vi "Main.vi"() -> ()   [LabVIEW 2015, in "Thermal Chamber Controller_DQMH.lvlib"]
doc: "This application is based on the Delacor QMH project template. Run this VI directly to test the module in stand alone mode. Run the module tester VI to test the module in external launch mode.\n\nThis example implements a Thermal Chamber Controller with a singleton Delacor QMH module.\n\n_____\nBased on Delacor QMH Project Template 3.0.\nReviewed and updated to match QMH Project Template 4.0.\n<b>Note:</b> This VI was modified by the <b>Validate DQMH Module</b> tool to upgrade it to the DQMH 3.0 implementation of the 'Show Diagram' message, which checks the password-protected status of the Main VI before showing the diagram.\n____\nDelacor QMH Thermal Chamber Examples 4.0.0.21\nCopyright (c) 2018, Delacor"
uses:
  Thermal Chamber Controller_DQMH.lvlib
  <vilib>/Delacor/Delacor QMH/Libraries/Module Admin_class/Delacor_lib_QMH_Module Admin.lvclass
  Module Data--cluster.ctl
  Heater State--enum.ctl
  Update Set Point Argument--cluster.ctl
  Update Ramp Rate Argument--cluster.ctl
  Update Heater State Argument--cluster.ctl
  Request and Wait for Status Argument--cluster.ctl
  Request and Wait for Status (Reply Payload)--cluster.ctl
  Stop Argument--cluster.ctl
  <vilib>/Delacor/Delacor QMH/Libraries/Module Admin_class/Delacor_lib_QMH_Module Admin.lvclass/Delacor_lib_QMH_Module Admin.ctl
  <vilib>/Delacor/Delacor QMH/Libraries/Module Admin_class/Delacor_lib_QMH_Get External Launch.vi
  <vilib>/Delacor/Delacor QMH/Libraries/Message Queue_class/Delacor_lib_QMH_Enqueue Message (Single).vi
  <vilib>/Utility/error.llb/Error Cluster From Error Code.vi
  <vilib>/ErrorRing/Error Ring.xnode
  <vilib>/Delacor/Delacor QMH/Libraries/Message Queue_class/Delacor_lib_QMH_Message Queue.lvclass
  Thermal Chamber Response Simulator/Thermal Chamber Response Simulator.lvlib
panel:
  in  "Enable Heater":bool
  in  "Disable Heater":bool
  in  "Ramp Rate (deg C / second)":dbl=1.0
  in  "Temperature Set Point (deg C)":dbl=22.0
  out "Heater State":bool
  out "Actual Temperature":dbl format="%.2f"
  out "Chamber Temperature Chart":T1(graph)
  in  "Simulate MHL Error":bool
  in  "Simulate EHL Error":bool
  out "error out":errorcluster
  in  "Module Admin":refnum<class "Delacor_lib_QMH_Module Admin.lvclass">
  out "Status":string
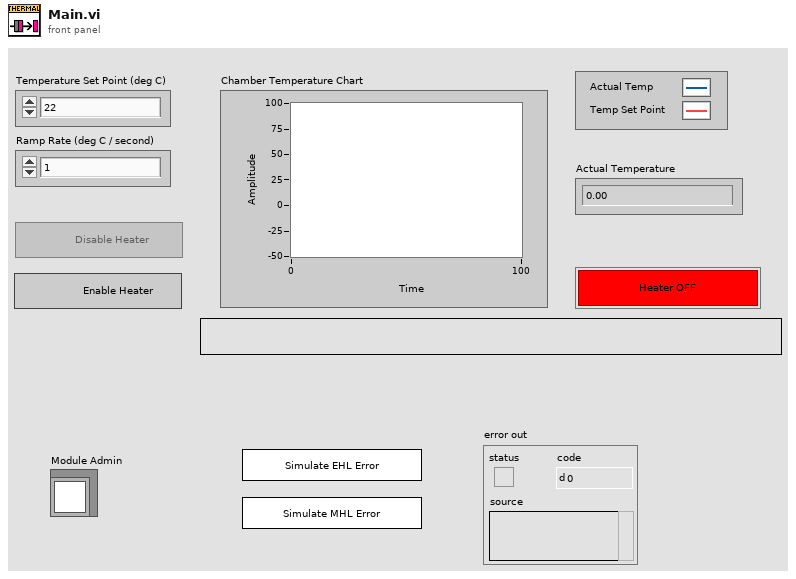
[diagram p1: front panel]
types:
  T1 = cluster{"Actual Temperature":dbl, "Required Temperature deg C":dbl}
  T2 = typedef "Thermal Chamber Controller_DQMH.lvlib/Request Events--cluster.ctl" = cluster{"Stop Module":refnum<user-event>, "Show Panel":refnum<user-event>, "Hide Panel":refnum<user-event>, "Get Module Execution Status":refnum<user-event>, "Show Diagram":refnum<user-event>, "Update Set Point":refnum<user-event>, "Update Ramp Rate":refnum<user-event>, "Update Heater State":refnum<user-event>, "Update Chamber Status":refnum<user-event>, "Request and Wait for Status":refnum<user-event>}
  T3 = typedef "Thermal Chamber Controller_DQMH.lvlib/Module Data--cluster.ctl" = cluster{"Status":string, "Temperature Set Point":dbl, "Temperature Ramp Rate":dbl, "Heater State":T4, "Disable Heater ref":refnum<vi>, "Enable Heater ref":refnum<vi>, "Temperature Set Point (deg C) ref":refnum<vi>, "Temperature Ramp Rate (Deg C / sec) ref":refnum<vi>}
  T4 = typedef "Thermal Chamber Controller_DQMH.lvlib/Heater State--enum.ctl" = enum16{"Heater Enabled", "Heater Disabled"}
  T5 = typedef "Thermal Chamber Controller_DQMH.lvlib/Update Set Point Argument--cluster.ctl" = cluster{"Temperature Set Point":dbl}
  T6 = typedef "Thermal Chamber Controller_DQMH.lvlib/Update Ramp Rate Argument--cluster.ctl" = cluster{"Temperature Ramp Rate":dbl}
  T7 = typedef "Thermal Chamber Controller_DQMH.lvlib/Update Heater State Argument--cluster.ctl" = cluster{"Heater State":T4}
  T8 = typedef "Thermal Chamber Controller_DQMH.lvlib/Request and Wait for Status Argument--cluster.ctl" = cluster{"Wait Notifier":refnum<notifier>}
  T9 = enum32{"invalid lock state", "Not Locked", "Locked (No Password)", "Password-protected"}
  T10 = typedef "Thermal Chamber Controller_DQMH.lvlib/Stop Argument--cluster.ctl" = cluster{"Origin":string, "Exit via Stop Module Req?":bool, "Wait for Module to stop?":bool}
  T11 = enum32{"Invalid", "Standard", "Closed", "Hidden", "Minimized", "Maximized"}
  T12 = typedef "Thermal Chamber Controller_DQMH.lvlib/Request and Wait for Status (Reply Payload)--cluster.ctl" = cluster{"Actual Temperature":dbl, "Temperature Set Point":dbl, "Temperature Ramp Rate":dbl, "Heater State":T4, "error":errorcluster}
  T13 = cluster{"Actual Temperature":dbl, "Temperature Set Point (deg C)":dbl}
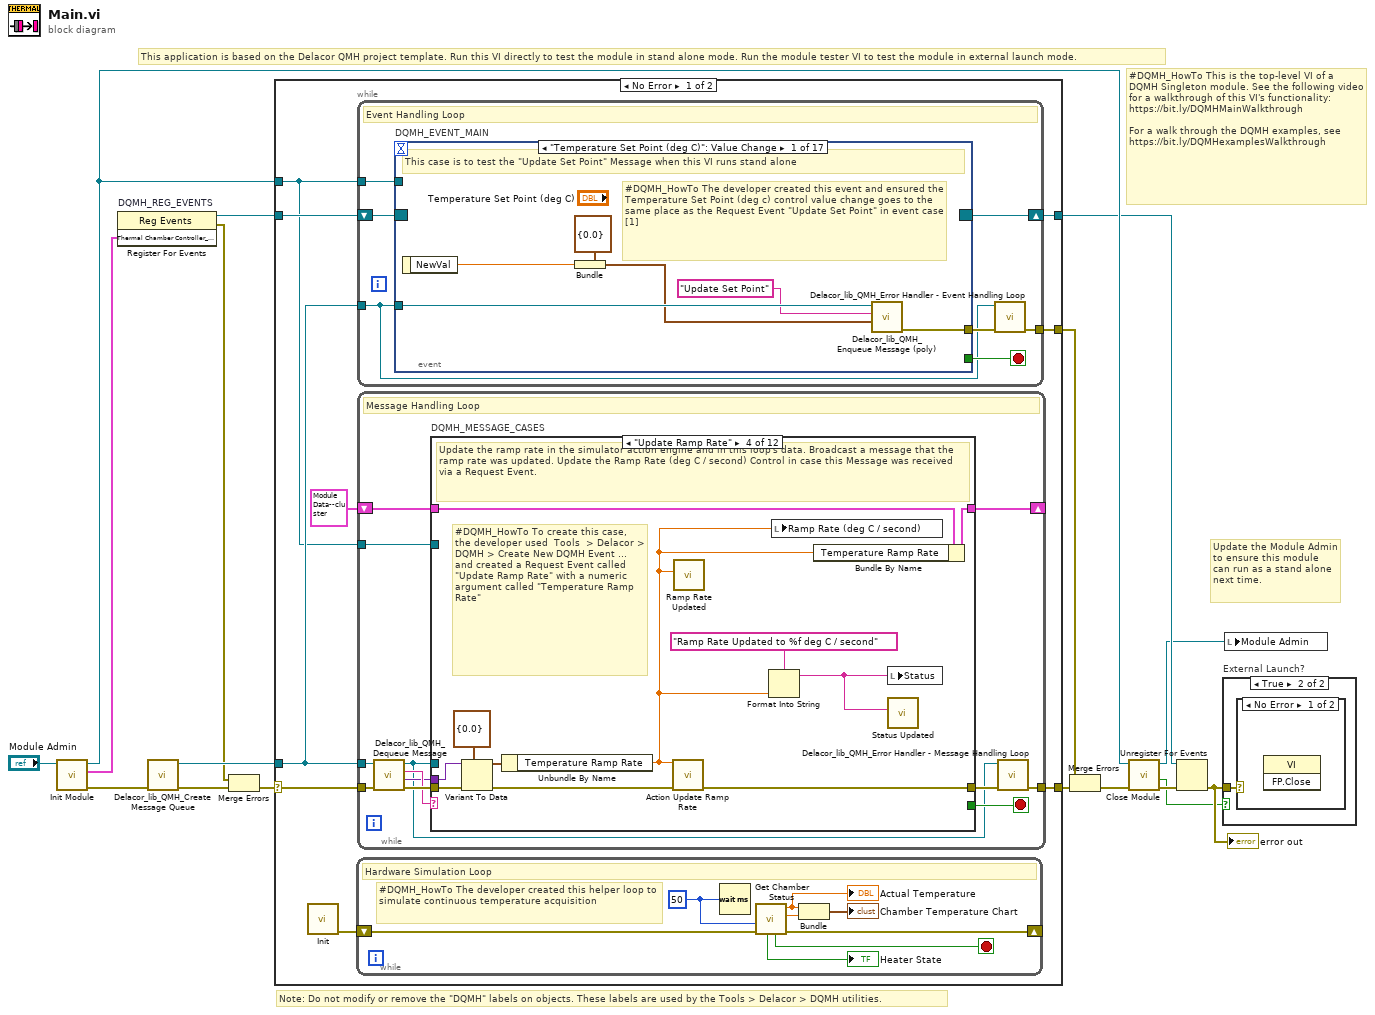
[diagram p0: block diagram]
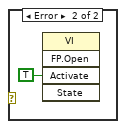
[diagram p3: hidden frame]
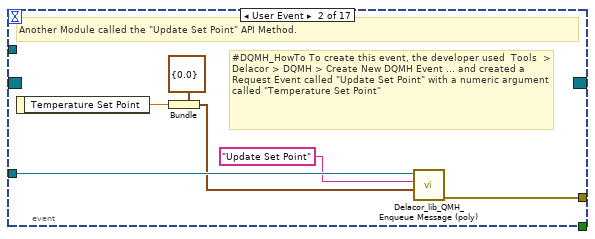
[diagram p4: hidden frame]
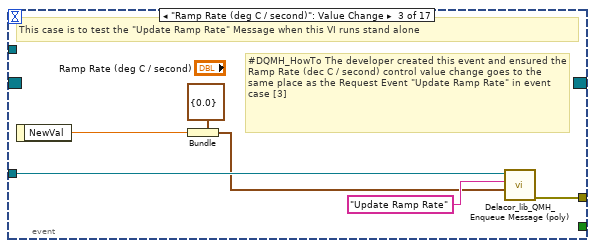
[diagram p5: hidden frame]
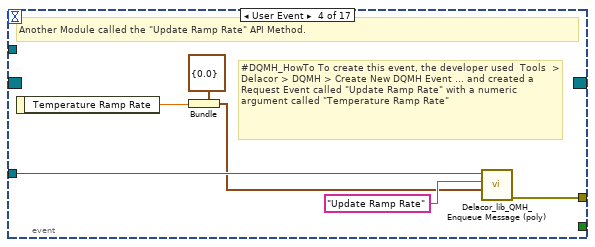
[diagram p6: hidden frame]
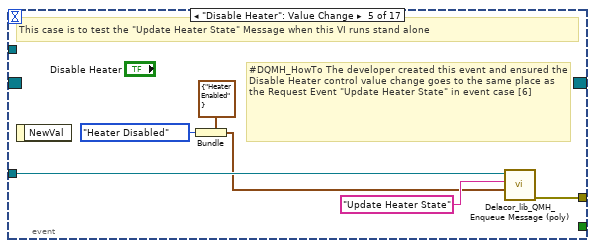
[diagram p7: hidden frame]
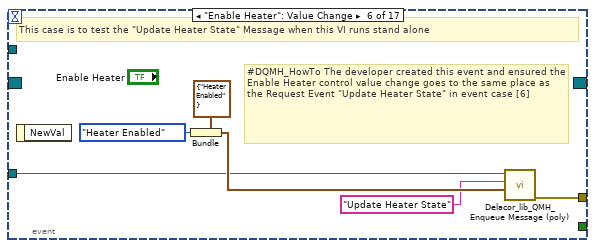
[diagram p8: hidden frame]
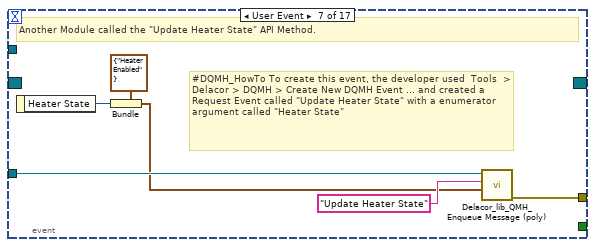
[diagram p9: hidden frame]
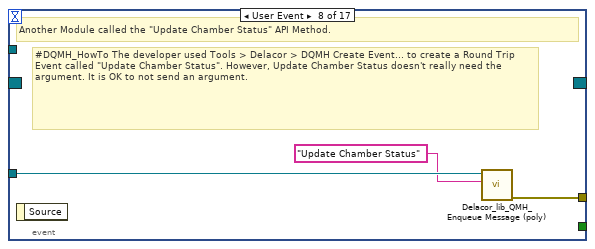
[diagram p10: hidden frame]
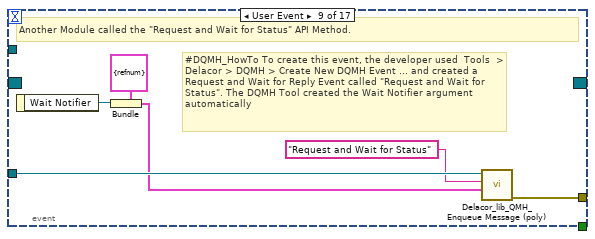
[diagram p11: hidden frame]
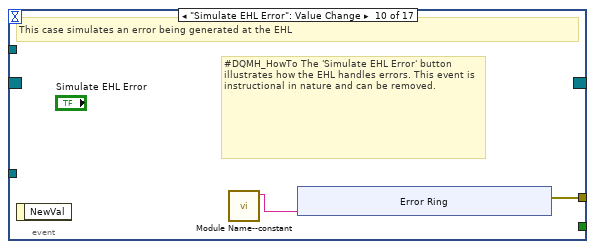
[diagram p12: hidden frame]
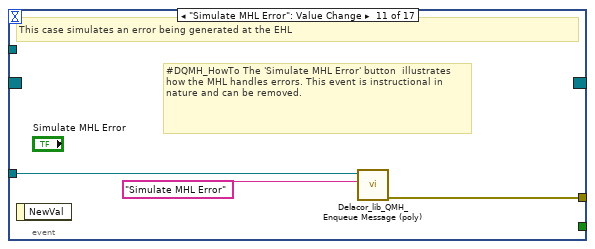
[diagram p13: hidden frame]
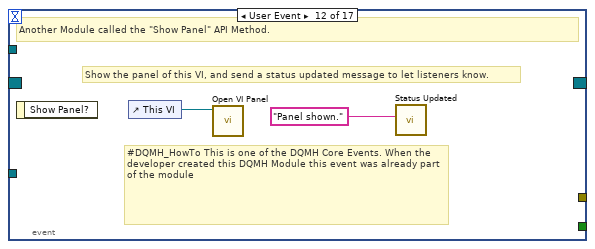
[diagram p14: hidden frame]
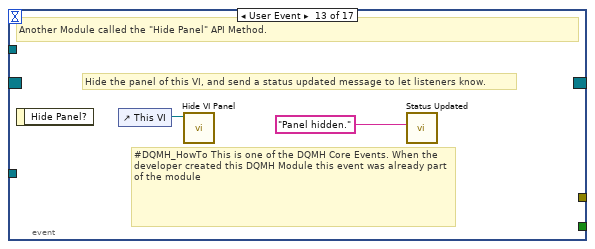
[diagram p15: hidden frame]
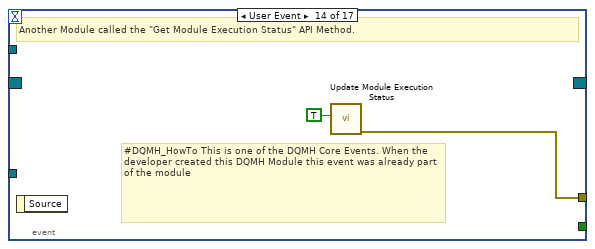
[diagram p16: hidden frame]
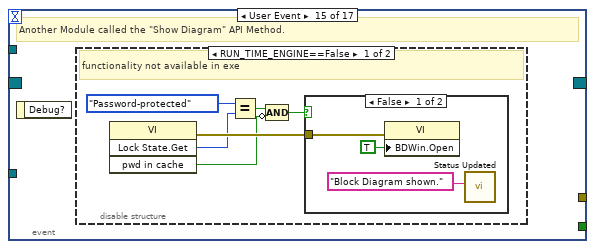
[diagram p17: hidden frame]
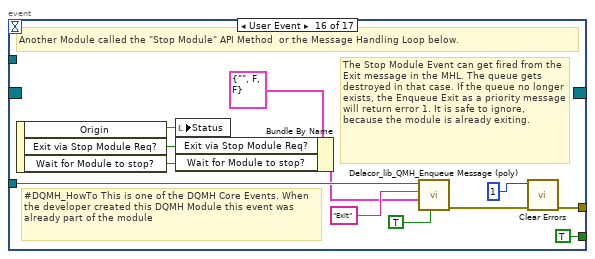
[diagram p20: hidden frame]
diagram:
  # "#DQMH_HowTo This is the top-level VI of a DQMH Singleton module. See the following video for a walkthrough of this VI's functionality: https://bit.ly/DQMHMainWalkthrough\n\nFor a walk through the DQMH examples, see https://bit.ly/DQMHexamplesWalkthrough"
  # "This application is based on the Delacor QMH project template. Run this VI directly to test the module in stand alone mode. Run the module tester VI to test the module in external launch mode."
  # "Note: Do not modify or remove the \"DQMH\" labels on objects. These labels are used by the Tools > Delacor > DQMH utilities."
  # "Update the Module Admin to ensure this module can run as a stand alone next time."
  n1 = call "Init Module.vi"("Singleton Module Admin in"="Module Admin") -> ("error out"=w15:errorcluster, "Thermal Chamber Controller_DQMH Request Events"=w12:T2, "Singleton Module Admin out"=w17:refnum<class "Delacor_lib_QMH_Module Admin.lvclass">)  [unwired: 8 in]
  n2 = register-events "DQMH_REG_EVENTS"(w12) -> (reference out=w13:refnum<event-registration>, error out=w1:errorcluster)  [unwired: 2 in]
  n3 = call <vilib>:"Delacor_lib_QMH_Create Message Queue.vi"("error in (no error)"=w15) -> ("error out"=w3:errorcluster, "Message Queue out"=w11:refnum<class "Delacor_lib_QMH_Message Queue.lvclass">)  [unwired: 9 in]
  n4 = Merge Errors(w1, w3) -> (w2:errorcluster)
  n5 = case shown="No Error" w2 {
    selector: w2 -> [w20 w314]
    tunnel: [w26 w314] -> w16
    tunnel: [w25 w319] -> w14
    tunnel: w13 -> [w23 w319]
    tunnel: w11 -> [w22 _]
    tunnel: [w21 _] -> w7
    tunnel: w17 -> [w19 w315]
    frame No Error {
      n6 = call "Init.vi"() -> ("error out"=w18:errorcluster)  [unwired: 11 in]
      n7 = while {
        shift-right: [w30] -> _
        shift-left: w18 -> [w33]
        stop <- w32 stop-if-true
        w34 = u32 50 ("millisecond multiple")
        # "#DQMH_HowTo The developer created this helper loop to simulate continuous temperature acquisition"
        # "Hardware Simulation Loop"
        n8 = Wait (ms)(milliseconds to wait=w34) -> ()  [unwired: 1 out]
        n9 = call "Get Chamber Status.vi"("error in (no error)"=w33, "Time Interval (ms)"=w34) -> ("error out"=w30:errorcluster, "Temperature Set Point (deg C)"=w31:dbl, "Actual Temperature"=w29:dbl, "Application Exit"=w32:bool, "Heater State"=→"Heater State":bool)  [unwired: 4 in, 1 out]
        "Actual Temperature" <- w29
        n10 = Bundle("Actual Temperature"=w29, "Temperature Set Point (deg C)"=w31) -> (→"Chamber Temperature Chart":T13)  [unwired: 1 in]
      }
      n11 = while {
        tunnel: w22 -> [w35]
        shift-right: [w40] -> w25
        shift-left: w23 -> [w41]
        tunnel: [w37] -> w21
        tunnel: w19 -> [w36]
        stop <- w38 stop-if-true
        # "Event Handling Loop"
        n12 = event "DQMH_EVENT_MAIN" shown="[0] \"Temperature Set Point (deg C)\": Value Change" {
          selector: w41 -> [_ _ _ _ _ _ _ _ _ _ _ _ _ _ _ _ _]
          dyn-events: [_ _ _ _ _ _ _ _ _ _ _ _ _ _ _ _ _] -> w40
          timeout: _ -> [_ _ _ _ _ _ _ _ _ _ _ _ _ _ _ _ _]
          tunnel: [_ _ _ _ _ _ _ _ _ _ _ _ _ _ _ TRUE ("Discard?") _] -> w38
          tunnel: w35 -> [w47 w53 w56 w65 w69 w74 w83 w86 w92 _ w104 _ _ _ _ w129 w132]
          tunnel: [w42 w49 w55 w61 w68 w73 w79 w84 w88 w94 w102 _ _ w110 _ w124 w134] -> w39
          tunnel: w36 -> [_ _ _ _ _ _ _ _ _ _ _ _ _ _ _ _ w135]
          event "Temperature Set Point (deg C)": Value Change {
            # "#DQMH_HowTo The developer created this event and ensured the Temperature Set Point (deg c) control value change goes to the same place as the Request Event \"Update Set Point\" in event case [1]"
            # "This case is to test the \"Update Set Point\" Message when this VI runs stand alone"
            n13 = event-data() -> ("NewVal"=w43:dbl)  [unwired: 1 in]
            n14 = Bundle(cluster=T5 {"Temperature Set Point"=0.0} ("Update Set Point Argument"), "Temperature Set Point"=w43) -> (w45:T5)
            n15 = call-poly <vilib>:"Delacor_lib_QMH_Enqueue Message (poly).vi"("Message Data"=w45, "Message"="Update Set Point", "Message Queue in"=w47) -> ("error out"=w42:errorcluster)  [unwired: 7 in, 1 out]
          }
          event User Event {
            # "#DQMH_HowTo To create this event, the developer used  Tools  > Delacor > DQMH > Create New DQMH Event ... and created a Request Event called \"Update Set Point\" with a numeric argument called \"Temperature Set Point\""
            # "Another Module called the \"Update Set Point\" API Method."
            n16 = event-data() -> ("Temperature Set Point"=w50:dbl)  [unwired: 1 in]
            n17 = Bundle(cluster=T5 {"Temperature Set Point"=0.0} ("Update Set Point Argument"), "Temperature Set Point"=w50) -> (w51:T5)
            n18 = call-poly <vilib>:"Delacor_lib_QMH_Enqueue Message (poly).vi"("Message Data"=w51, "Message"="Update Set Point", "Message Queue in"=w53) -> ("error out"=w49:errorcluster)  [unwired: 7 in, 1 out]
          }
          event "Ramp Rate (deg C / second)": Value Change {
            # "#DQMH_HowTo The developer created this event and ensured the Ramp Rate (dec C / second) control value change goes to the same place as the Request Event \"Update Ramp Rate\" in event case [3]"
            # "This case is to test the \"Update Ramp Rate\" Message when this VI runs stand alone"
            n19 = event-data() -> ("NewVal"=w57:dbl)  [unwired: 1 in]
            n20 = Bundle(cluster=T6 {"Temperature Ramp Rate"=0.0} ("Update Ramp Rate Argument"), "Temperature Ramp Rate"=w57) -> (w54:T6)
            n21 = call-poly <vilib>:"Delacor_lib_QMH_Enqueue Message (poly).vi"("Message Data"=w54, "Message"="Update Ramp Rate", "Message Queue in"=w56) -> ("error out"=w55:errorcluster)  [unwired: 7 in, 1 out]
          }
          event User Event {
            # "#DQMH_HowTo To create this event, the developer used  Tools  > Delacor > DQMH > Create New DQMH Event ... and created a Request Event called \"Update Ramp Rate\" with a numeric argument called \"Temperature Ramp Rate\""
            # "Another Module called the \"Update Ramp Rate\" API Method."
            n22 = event-data() -> ("Temperature Ramp Rate"=w60:dbl)  [unwired: 1 in]
            n23 = Bundle(cluster=T6 {"Temperature Ramp Rate"=0.0} ("Update Ramp Rate Argument"), "Temperature Ramp Rate"=w60) -> (w62:T6)
            n24 = call-poly <vilib>:"Delacor_lib_QMH_Enqueue Message (poly).vi"("Message Data"=w62, "Message"="Update Ramp Rate", "Message Queue in"=w65) -> ("error out"=w61:errorcluster)  [unwired: 7 in, 1 out]
          }
          event "Disable Heater": Value Change {
            # "#DQMH_HowTo The developer created this event and ensured the Disable Heater control value change goes to the same place as the Request Event \"Update Heater State\" in event case [6]"
            # "This case is to test the \"Update Heater State\" Message when this VI runs stand alone"
            n25 = event-data() -> ()  [unwired: 1 in, 1 out]
            n26 = Bundle(cluster=T7 {"Heater State"=enum."Heater Enabled"} ("Update Heater State Argument"), "Heater State"=Heater_State--enum."Heater Disabled") -> (w67:T7)
            n27 = call-poly <vilib>:"Delacor_lib_QMH_Enqueue Message (poly).vi"("Message Data"=w67, "Message"="Update Heater State", "Message Queue in"=w69) -> ("error out"=w68:errorcluster)  [unwired: 7 in, 1 out]
          }
          event "Enable Heater": Value Change {
            # "#DQMH_HowTo The developer created this event and ensured the Enable Heater control value change goes to the same place as the Request Event \"Update Heater State\" in event case [6]"
            # "This case is to test the \"Update Heater State\" Message when this VI runs stand alone"
            n28 = event-data() -> ()  [unwired: 1 in, 1 out]
            n29 = Bundle(cluster=T7 {"Heater State"=enum."Heater Enabled"} ("Update Heater State Argument"), "Heater State"=Heater_State--enum."Heater Enabled") -> (w77:T7)
            n30 = call-poly <vilib>:"Delacor_lib_QMH_Enqueue Message (poly).vi"("Message Data"=w77, "Message"="Update Heater State", "Message Queue in"=w74) -> ("error out"=w73:errorcluster)  [unwired: 7 in, 1 out]
          }
          event User Event {
            # "#DQMH_HowTo To create this event, the developer used  Tools  > Delacor > DQMH > Create New DQMH Event ... and created a Request Event called \"Update Heater State\" with a enumerator argument called \"Heater State\""
            # "Another Module called the \"Update Heater State\" API Method."
            n31 = event-data() -> ("Heater State"=w78:T4)  [unwired: 1 in]
            n32 = Bundle(cluster=T7 {"Heater State"=enum."Heater Enabled"} ("Update Heater State Argument"), "Heater State"=w78) -> (w80:T7)
            n33 = call-poly <vilib>:"Delacor_lib_QMH_Enqueue Message (poly).vi"("Message Data"=w80, "Message"="Update Heater State", "Message Queue in"=w83) -> ("error out"=w79:errorcluster)  [unwired: 7 in, 1 out]
          }
          event User Event {
            # "#DQMH_HowTo The developer used Tools > Delacor > DQMH Create Event... to create a Round Trip Event called \"Update Chamber Status\". However, Update Chamber Status doesn't really need the argument. It is OK to not send an argument."
            # "Another Module called the \"Update Chamber Status\" API Method."
            n34 = event-data() -> ()  [unwired: 1 in, 1 out]
            n35 = call-poly <vilib>:"Delacor_lib_QMH_Enqueue Message (poly).vi"("Message"="Update Chamber Status", "Message Queue in"=w86) -> ("error out"=w84:errorcluster)  [unwired: 8 in, 1 out]
          }
          event User Event {
            # "#DQMH_HowTo To create this event, the developer used  Tools  > Delacor > DQMH > Create New DQMH Event ... and created a Request and Wait for Reply Event called \"Request and Wait for Status\". The DQMH Tool created the Wait Notifier argument automatically"
            # "Another Module called the \"Request and Wait for Status\" API Method."
            n36 = event-data() -> ("Wait Notifier"=w87:refnum<notifier>)  [unwired: 1 in]
            n37 = Bundle(cluster=T8 {"Wait Notifier"=refnum} ("Request and Wait for Status Argument"), "Wait Notifier"=w87) -> (w89:T8)
            n38 = call-poly <vilib>:"Delacor_lib_QMH_Enqueue Message (poly).vi"("Message Data"=w89, "Message"="Request and Wait for Status", "Message Queue in"=w92) -> ("error out"=w88:errorcluster)  [unwired: 7 in, 1 out]
          }
          event "Simulate EHL Error": Value Change {
            # "#DQMH_HowTo The 'Simulate EHL Error' button  illustrates how the EHL handles errors. This event is instructional in nature and can be removed."
            # "This case simulates an error being generated at the EHL"
            n39 = event-data() -> ()  [unwired: 1 in, 1 out]
            n40 = call "Module Name--constant.vi"() -> ("Module Name"=w93:string)  [unwired: 11 in]
            n41 = xnode ("Error Ring")("parameter 0"=w93) -> ("error out"=w94:errorcluster)
          }
          event "Simulate MHL Error": Value Change {
            # "#DQMH_HowTo The 'Simulate MHL Error' button  illustrates how the MHL handles errors. This event is instructional in nature and can be removed."
            # "This case simulates an error being generated at the EHL"
            n42 = event-data() -> ()  [unwired: 1 in, 1 out]
            n43 = call-poly <vilib>:"Delacor_lib_QMH_Enqueue Message (poly).vi"("Message"="Simulate MHL Error", "Message Queue in"=w104) -> ("error out"=w102:errorcluster)  [unwired: 8 in, 1 out]
          }
          event User Event {
            # "#DQMH_HowTo This is one of the DQMH Core Events. When the developer created this DQMH Module this event was already part of the module"
            # "Show the panel of this VI, and send a status updated message to let listeners know."
            # "Another Module called the \"Show Panel\" API Method."
            n44 = event-data() -> ()  [unwired: 1 in, 1 out]
            n45 = control-ref of="This VI"() -> (w105:refnum<vi>)
            n46 = call "Open VI Panel.vi"("VI"=w105) -> ()  [unwired: 10 in, 1 out]
            n47 = call "Status Updated.vi"("Status"="Panel shown." ("format string")) -> ()  [unwired: 10 in, 1 out]
          }
          event User Event {
            # "#DQMH_HowTo This is one of the DQMH Core Events. When the developer created this DQMH Module this event was already part of the module"
            # "Hide the panel of this VI, and send a status updated message to let listeners know."
            # "Another Module called the \"Hide Panel\" API Method."
            n48 = event-data() -> ()  [unwired: 1 in, 1 out]
            n49 = control-ref of="This VI"() -> (w107:refnum<vi>)
            n50 = call "Hide VI Panel.vi"("VI"=w107) -> ()  [unwired: 10 in, 1 out]
            n51 = call "Status Updated.vi"("Status"="Panel hidden." ("format string")) -> ()  [unwired: 10 in, 1 out]
          }
          event User Event {
            # "#DQMH_HowTo This is one of the DQMH Core Events. When the developer created this DQMH Module this event was already part of the module"
            # "Another Module called the \"Get Module Execution Status\" API Method."
            n52 = event-data() -> ()  [unwired: 1 in, 1 out]
            n53 = call "Update Module Execution Status.vi"("Running?"=TRUE) -> ("error out"=w110:errorcluster)  [unwired: 10 in]
          }
          event User Event {
            # "Another Module called the \"Show Diagram\" API Method."
            n54 = event-data() -> ()  [unwired: 1 in, 1 out]
            n55 = disable-structure "Conditional Disable Structure" shown="RUN_TIME_ENGINE==False" {
              frame condition #0 (active) {
                # "functionality not available in exe"
                n56 = invoke on="Invoke Node" class="VI" method="Lock State.Get"() -> (error out=w116:errorcluster, "Get Lock State"=w115:T9, "pwd in cache"=w112:bool)  [unwired: 4 in, 1 out]
                n57 = Equal?(x=T9."Password-protected", y=w115) -> (x = y?=w113:bool)
                n58 = Compound Arithmetic op=AND(w113, invert w112) -> (w111:bool)
                n59 = case shown="False" w111 {
                  tunnel: w116 -> [w118 _]
                  frame False {
                    n60 = property on="Property Node" class="VI"(error in=w118, "BDWin.Open"=TRUE ("Block Diagram Window:Open")) -> ()  [unwired: 1 in, 2 out]
                    n61 = call "Status Updated.vi"("Status"="Block Diagram shown." ("format string")) -> ()  [unwired: 10 in, 1 out]
                  }
                  frame True {
                    # "Password-protected VI, and the password is not in the cache. Do not show the diagram."
                  }
                }
              }
              frame condition #1 {
                # "#DQMH_HowTo This is one of the DQMH Core Events. When the developer created this DQMH Module this event was already part of the module"
              }
            }
          }
          event User Event {
            # "#DQMH_HowTo This is one of the DQMH Core Events. When the developer created this DQMH Module this event was already part of the module"
            # "The Stop Module Event can get fired from the Exit message in the MHL. The queue gets destroyed in that case. If the queue no longer exists, the Enqueue Exit as a priority message will return error 1. It is safe to ignore, because the module is already exiting."
            # "Another Module called the \"Stop Module\" API Method  or the Message Handling Loop below."
            n62 = event-data() -> ("Origin"=w128:string, "Exit via Stop Module Req?"=w122:bool, "Wait for Module to stop?"=w121:bool)  [unwired: 1 in]
            n63 = local write "Status"(w128) -> ()
            n64 = Bundle By Name(cluster=T10 {"Origin"="", "Exit via Stop Module Req?"=FALSE, "Wait for Module to stop?"=FALSE} ("Stop Argument"), "Exit via Stop Module Req?"=w122, "Wait for Module to stop?"=w121) -> (w120:T10)
            n65 = call-poly <vilib>:"Delacor_lib_QMH_Enqueue Message (poly).vi"("Priority Message? (F)"=TRUE, "Message Data"=w120, "Message"="Exit", "Message Queue in"=w129) -> ("error out"=w125:errorcluster)  [unwired: 6 in, 1 out]
            n66 = call <vilib>:"Clear Errors.vi"("error in (no error)"=w125, "specific error code to clear (0: all)"=1) -> ("error out"=w124:errorcluster)  [unwired: 4 in, 1 out]
          }
          event Panel Close? {
            w136 = TRUE  # Discard the event so the Exit message has a chance to run.
            # "#DQMH_HowTo When the developer created this DQMH Module this event was already part of the module"
            # "Send the Exit message if the user closes the panel of the VI."
            n67 = event-data() -> ()  [unwired: 1 in, 1 out]
            n68 = property on="Property Node" class="Module Admin"(reference=w135) -> ("Accessors:External Launch"=w133:bool)  [unwired: 1 in, 2 out]
            n69 = case shown="True" w133 {
              tunnel: w132 -> [_ w141]
              tunnel: [_ w140] -> w134
              frame True {
                # "If externally launched, clicking the 'X' hides the panel, but doesn't close it."
                n70 = control-ref of="This VI"() -> (w137:refnum<vi>)
                n71 = call "Hide VI Panel.vi"("VI"=w137) -> ()  [unwired: 10 in, 1 out]
              }
              frame False {
                # "If run as a stand-alone VI, clicking the panel 'X' stops the VI."
                n72 = call-poly <vilib>:"Delacor_lib_QMH_Enqueue Message (poly).vi"("Priority Message? (F)"=TRUE, "Message"="Exit", "Message Queue in"=w141) -> ("error out"=w140:errorcluster)  [unwired: 7 in, 1 out]
              }
            }
            n73 = event-data ("Event Filter Node")("Discard?"=w136) -> ()  [unwired: 1 in, 1 out]
          }
        }
        n74 = call-dynamic "Delacor_lib_QMH_Error Handler - Event Handling Loop.vi"("error in (no error)"=w39, "Message Queue in"=w35) -> ("dup error in"=w37:errorcluster)  [unwired: 8 in, 1 out]
      }
      n75 = while {
        tunnel: w22 -> [w145]
        shift-right: [w151] -> _
        shift-left: T3 {"Status"="", "Temperature Set Point"=0.0, "Temperature Ramp Rate"=0.0, "Heater State"=enum."Heater Enabled", "Disable Heater ref"=refnum, "Enable Heater ref"=refnum, "Temperature Set Point (deg C) ref"=refnum, "Temperature Ramp Rate (Deg C / sec) ref"=refnum} ("Data Cluster") -> [w152]
        tunnel: w20 -> [w149]
        tunnel: [w143] -> w26
        tunnel: w19 -> [w142]
        stop <- w150 stop-if-true
        # "Message Handling Loop"
        n76 = call-dynamic "Delacor_lib_QMH_Dequeue Message.vi"("error in (no error)"=w149, "Message Queue in"=w145) -> ("error out"=w148:errorcluster, "Message Data"=w146:variant, "Message"=w147:string, "Message Queue out"=w144:refnum<class "Delacor_lib_QMH_Message Queue.lvclass">)  [unwired: 6 in]
        n77 = case "DQMH_MESSAGE_CASES" shown="\"Update Ramp Rate\"" w147 {
          selector: w147 -> [_ _ _ _ _ _ _ _ _ _ _ w301]
          tunnel: w144 -> [_ _ _ _ _ _ _ _ _ w270 w297 _]
          tunnel: w148 -> [w171 w184 w195 w206 w222 w225 w238 w255 w260 w277 w299 _]
          tunnel: [w165 w182 w185 w198 w218 w226 w240 w253 w258 w271 w293 w302] -> w153
          tunnel: w152 -> [w170 w183 w190 w202 w215 w233 w252 w254 w259 w276 w296 w303]
          tunnel: [w169 w183 w189 w201 w207 w233 w252 w254 w259 w276 w296 w303] -> w151
          tunnel: [_ _ _ _ _ _ _ _ _ _ w295 _] -> w150
          tunnel: w146 -> [_ _ w188 w200 w221 _ w251 _ _ w275 w292 _]
          tunnel: w142 -> [w172 _ _ _ _ _ _ _ _ w269 w286 _]
          frame "Initialize" {
            w157 = Heater_State--enum."Heater Disabled" ("Heater State")
            w154 = "Initial Message" ("Initial Message")
            # "Initialize - Any operation that needs to be done before the module can receive messages. Synchronize Caller Events.vi will inform Start Module.vi that the module has launched and is ready to receive messages. Module Did Init.vi will broadcast that the module initialized."
            n78 = call "Synchronize Caller Events.vi"("error in (no error)"=w171, "Singleton Module Admin in"=w172) -> ("error out"=w166:errorcluster, "Singleton Module Admin out"=w164:refnum<class "Delacor_lib_QMH_Module Admin.lvclass">)  [unwired: 8 in]
            n79 = property on="Property Node" class="Module Admin"(reference=w164) -> ("Accessors:External Launch"=w176:bool)  [unwired: 1 in, 2 out]
            n80 = control-ref of="Disable Heater"() -> (w159:refnum<vi>)
            n81 = control-ref of="Enable Heater"() -> (w158:refnum<vi>)
            n82 = control-ref of="Ramp Rate (deg C / second)"() -> (w160:refnum<vi>)
            n83 = control-ref of="Temperature Set Point (deg C)"() -> (w161:refnum<vi>)
            n84 = call "Heater State Controls Interlocks.vi"("Enable Heater ref in"=w158, "Heater State"=w157, "Disable Heater ref in"=w159) -> ("Enable Heater ref out"=w155:refnum<vi>, "Disable Heater ref out"=w156:refnum<vi>)  [unwired: 7 in]
            n85 = Select(t=T11."Hidden" ("State"), s=w176, f=T11."Standard" ("State")) -> (s? t:f=w173:T11)
            n86 = call "Module Name--constant.vi"() -> ("Module Name"=w181:string)  [unwired: 11 in]
            n87 = Bundle By Name(cluster=w170, "Status"=w154, "Temperature Set Point"=22.0, "Temperature Ramp Rate"=1.0, "Temperature Ramp Rate (Deg C / sec) ref"=w160, "Temperature Set Point (deg C) ref"=w161, "Disable Heater ref"=w156, "Enable Heater ref"=w155, "Heater State"=w157) -> (w169:T3)
            n88 = property on="Property Node" class="VI"("Front Panel.Title"=w181) -> (reference out=w179:refnum<vi>, error out=w180:errorcluster)  [unwired: 2 in]
            n89 = call "Module Name--constant.vi"() -> ("Module Name"=w167:string)  [unwired: 11 in]
            n90 = invoke on="Invoke Node" class="VI" method="FP.Open"(reference=w179, error in=w180, "State"=w173) -> (reference out=w178:refnum<vi>, error out=w177:errorcluster)  [unwired: 2 in, 3 out]
            n91 = call "Module Did Init.vi"("error in (no error)"=w166, "Initialized?"=TRUE, "Origin"=w167) -> ("error out"=w165:errorcluster)  [unwired: 8 in]
            n92 = invoke on="Invoke Node" class="VI" method="FP.Center"(reference=w178, error in=w177) -> ()  [unwired: 1 in, 3 out]
            "Status" <- w154
          }
          frame "--- Thermal Chamber Control ---" {
            # "Separator - Following cases update the Thermal Chamber control."
            n93 = Merge Errors(w184) -> (w182:errorcluster)
          }
          frame "Update Set Point" {
            # "#DQMH_HowTo To create this case, the developer used  Tools  > Delacor > DQMH > Create New DQMH Event ... and created a Request Event called \"Update Set Point\" with a numeric argument called \"Temperature Set Point\""
            # "Update the set point in the simulator action engine and in this loop's data. Broadcast a message that the set point was updated. Update the Temperature Set Point (deg C) Control in case this Message was received via a Request Event."
            n94 = Variant To Data(error in=w195, type=T5 {"Temperature Set Point"=0.0} ("Update Set Point Argument"), Variant=w188) -> (data=w193:T5, error out=w191:errorcluster)
            n95 = Unbundle By Name(w193) -> ("Temperature Set Point"=w187:dbl)
            n96 = call "Action Update Set Point.vi"("error in (no error)"=w191, "Temperature Set Point"=w187) -> ("error out"=w185:errorcluster)  [unwired: 9 in]
            n97 = call "Set Point Updated.vi"("Temperature Set Point"=w187) -> ()  [unwired: 10 in, 1 out]
            n98 = Format Into String(format string="Set Point Updated to %f deg C", w187) -> (resulting string=w186:string)  [unwired: 2 in, 1 out]
            n99 = local write "Temperature Set Point (deg C)"(w187) -> ()
            n100 = Bundle By Name(cluster=w190, "Temperature Set Point"=w187) -> (w189:T3)
            n101 = local write "Status"(w186) -> ()
            n102 = call "Status Updated.vi"("Status"=w186) -> ()  [unwired: 10 in, 1 out]
          }
          frame "Update Ramp Rate" {
            # "#DQMH_HowTo To create this case, the developer used  Tools  > Delacor > DQMH > Create New DQMH Event ... and created a Request Event called \"Update Ramp Rate\" with a numeric argument called \"Temperature Ramp Rate\""
            # "Update the ramp rate in the simulator action engine and in this loop's data. Broadcast a message that the ramp rate was updated. Update the Ramp Rate (deg C / second) Control in case this Message was received via a Request Event."
            n103 = Variant To Data(error in=w206, type=T6 {"Temperature Ramp Rate"=0.0} ("Update Ramp Rate Argument"), Variant=w200) -> (data=w204:T6, error out=w199:errorcluster)
            n104 = Unbundle By Name(w204) -> ("Temperature Ramp Rate"=w197:dbl)
            n105 = call "Action Update Ramp Rate.vi"("error in (no error)"=w199, "Temperature Ramp Rate"=w197) -> ("error out"=w198:errorcluster)  [unwired: 9 in]
            n106 = call "Ramp Rate Updated.vi"("Temperature Ramp Rate"=w197) -> ()  [unwired: 10 in, 1 out]
            n107 = Format Into String(format string="Ramp Rate Updated to %f deg C / second", w197) -> (resulting string=w196:string)  [unwired: 2 in, 1 out]
            n108 = local write "Ramp Rate (deg C / second)"(w197) -> ()
            n109 = Bundle By Name(cluster=w202, "Temperature Ramp Rate"=w197) -> (w201:T3)
            n110 = local write "Status"(w196) -> ()
            n111 = call "Status Updated.vi"("Status"=w196) -> ()  [unwired: 10 in, 1 out]
          }
          frame "Update Heater State" {
            # "#DQMH_HowTo To create this case, the developer used  Tools  > Delacor > DQMH > Create New DQMH Event ... and created a Request Event called \"Update Heater State\" with an enumerator argument called \"Heater State\""
            # "Update Heater controls interlocks depending on current Heater State."
            # "Update the heater state in the simulator action engine and in this loop's data. Broadcast a message that the heater state was updated. Update the Heater State controls in case this Message was received via a Request Event."
            n112 = Variant To Data(error in=w222, type=T7 {"Heater State"=enum."Heater Enabled"} ("Update Heater State Argument"), Variant=w221) -> (data=w219:T7, error out=w214:errorcluster)
            n113 = Unbundle By Name(w215) -> ("Temperature Set Point"=w217:dbl, "Temperature Ramp Rate"=w216:dbl)
            n114 = Unbundle By Name(w219) -> ("Heater State"=w212:T4)
            n115 = Bundle By Name(cluster=w215, "Heater State"=w212) -> (w207:T3)
            n116 = call "Heater State Updated.vi"("Heater State"=w212) -> ()  [unwired: 10 in, 1 out]
            n117 = Format Into String(format string="Heater State Updated to: %s", w212) -> (resulting string=w211:string)  [unwired: 2 in, 1 out]
            n118 = call "Action Update Heater State.vi"("error in (no error)"=w214, "Heater State"=w212, "Temperature Ramp Rate"=w216, "Temperature Set Point"=w217) -> ("error out"=w218:errorcluster)  [unwired: 7 in]
            n119 = local write "Status"(w211) -> ()
            n120 = call "Status Updated.vi"("Status"=w211) -> ()  [unwired: 10 in, 1 out]
            n121 = Unbundle By Name(w207) -> ("Disable Heater ref"=w210:refnum<vi>, "Heater State"=w209:T4, "Enable Heater ref"=w208:refnum<vi>)
            n122 = call "Heater State Controls Interlocks.vi"("Enable Heater ref in"=w208, "Heater State"=w209, "Disable Heater ref in"=w210) -> ()  [unwired: 7 in, 2 out]
          }
          frame "Update Chamber Status" {
            # "#DQMH_HowTo To create this case, the developer used Tools > Delacor > DQMH Create Event... to create a Round Trip Event called \"Update Chamber Status\". However, Update Chamber Status doesn't really need the argument. It is OK to not send an argument."
            # "Get the status from the simulator action engine, and broadcast it. Since this message originated from the \"Update Chamber Status\" request, this is an example of a Round Trip DQMH event."
            n123 = call "Status Updated.vi"("error in (no error)"=w225, "Status"="Request received to update Chamber Status. Reply will be sent via broadcast.") -> ("error out"=w224:errorcluster)  [unwired: 9 in]
            n124 = call "Get Chamber Status.vi"("error in (no error)"=w224) -> ("error out"=w229:errorcluster, "Ramp Rate (deg C / second)"=w230:dbl, "Temperature Set Point (deg C)"=w231:dbl, "Actual Temperature"=w232:dbl, "Heater State"=w228:bool)  [unwired: 5 in, 1 out]
            n125 = call "Convert Shutdown Furnace to Heater State Enum.vi"("Shutdown Furnace?"=w228) -> ("Heater State"=w227:T4)  [unwired: 10 in]
            n126 = call "Chamber Status Updated.vi"("Heater State"=w227, "error in (no error)"=w229, "Temperature Ramp Rate"=w230, "Temperature Set Point"=w231, "Actual Temperature"=w232) -> ("error out"=w226:errorcluster)  [unwired: 6 in]
          }
          frame "Request and Wait for Status" {
            # "#DQMH_HowTo To create this case, the developer used  Tools  > Delacor > DQMH > Create New DQMH Event ... and created a Request and Wait for Reply Event called \"Request and Wait for Status\". The DQMH Tool created the Wait Notifier argument automatically"
            # "Get the status from the simulator action engine, and send it to a waiting notifier. Since this message originated from the \"Request and Wait for Status\" request, this is an example of a Request and Wait for Reply DQMH event."
            n127 = Variant To Data(error in=w238, type=T8 {"Wait Notifier"=refnum} ("Request and Wait for Status Argument"), Variant=w251) -> (data=w249:T8, error out=w237:errorcluster)
            n128 = Unbundle By Name(w249) -> ("Wait Notifier"=w248:refnum<notifier>)
            n129 = call "Status Updated.vi"("error in (no error)"=w237, "Status"="Request received to update Chamber Status. Reply will be sent immediately via Request VI's output") -> ("error out"=w236:errorcluster)  [unwired: 9 in]
            n130 = call "Get Chamber Status.vi"("error in (no error)"=w236) -> ("error out"=w235:errorcluster, "Ramp Rate (deg C / second)"=w245:dbl, "Temperature Set Point (deg C)"=w246:dbl, "Actual Temperature"=w247:dbl, "Heater State"=w242:bool)  [unwired: 5 in, 1 out]
            n131 = call "Convert Shutdown Furnace to Heater State Enum.vi"("Shutdown Furnace?"=w242) -> ("Heater State"=w241:T4)  [unwired: 10 in]
            n132 = Bundle By Name(cluster=T12 {"Actual Temperature"=0.0, "Temperature Set Point"=0.0, "Temperature Ramp Rate"=0.0, "Heater State"=enum."Heater Enabled", "error"={"status"=FALSE, "code"=0, "source"=""}} ("notification"), "Actual Temperature"=w247, "Temperature Set Point"=w246, "Temperature Ramp Rate"=w245, "Heater State"=w241, "error"=w235) -> (w243:T12)
            n133 = Send Notification(notification=w243, notifier=w248) -> (error out=w239:errorcluster)  [unwired: 1 in, 1 out]
            n134 = Merge Errors(w235, w239) -> (w240:errorcluster)
          }
          frame "---Exit and Error Handling---" {
            # "Separator - the following cases handle errors and exit messages."
            n135 = Merge Errors(w255) -> (w253:errorcluster)
          }
          frame "Simulate MHL Error" {
            # "#DQMH_HowTo The 'Simulate MHL Error' button  illustrates how the MHL handles errors. This event is instructional in nature and can be removed."
            # "Simulate an error occurring at the MHL"
            n136 = call "Module Name--constant.vi"() -> ("Module Name"=w257:string)  [unwired: 11 in]
            n137 = xnode ("Error Ring")("parameter 0"=w257) -> ("error out"=w256:errorcluster)
            n138 = Merge Errors(w260, w256) -> (w258:errorcluster)
          }
          frame "Error" {
            # "#DQMH_HowTo When the developer created this DQMH Module this case was already part of the module"
            # "Error - Check the error message data and respond accordingly. This message is sent by the \"Error Handler\" VIs at the end of each loop in this application."
            n139 = property on="Property Node" class="Module Admin"(reference=w269) -> ("Accessors:External Launch"=w268:bool)  [unwired: 1 in, 2 out]
            n140 = Variant To Data(error in=w277, type=errorcluster {"status"=FALSE, "code"=0, "source"=""} ("error constant"), Variant=w275) -> (data=w278:errorcluster, error out=w273:errorcluster)
            n141 = call "Error Reported.vi"("Error"=w278) -> ()  [unwired: 10 in, 1 out]
            n142 = case shown="False" w268 {
              tunnel: [w283 _] -> w272
              tunnel: w270 -> [w282 _]
              tunnel: w278 -> [w279 _]
              frame False {
                # "If the module is running standalone, then pop up an error dialog and call the \"Exit\" message."
                n143 = call <vilib>:"Simple Error Handler.vi"("error in (no error)"=w279) -> ()  [unwired: 4 in, 5 out]
                n144 = call-poly <vilib>:"Delacor_lib_QMH_Enqueue Message (poly).vi"("Priority Message? (F)"=TRUE, "Message"="Exit", "Message Queue in"=w282) -> ("error out"=w283:errorcluster)  [unwired: 7 in, 1 out]
              }
              frame True {
                # "If the module was launched externally, calling the Error Reported broadcast VI is the only action performed by the \"Error\" message. The module's caller can then process the error appropriately."
              }
            }
            n145 = Merge Errors(w273, w272) -> (w271:errorcluster)
          }
          frame "Exit" {
            w290 = 91  # 91: not all Exit messages will have an argument
            w295 = TRUE  # Stop the VI
            # "#DQMH_HowTo When the developer created this DQMH Module this case was already part of the module"
            # "Release the message queue reference"
            # "Exit - Exit the application."
            n146 = Variant To Data(error in=w299, type=T10 {"Origin"="", "Exit via Stop Module Req?"=FALSE, "Wait for Module to stop?"=FALSE} ("Stop Argument"), Variant=w292) -> (data=w288:T10, error out=w291:errorcluster)
            n147 = call <vilib>:"Clear Errors.vi"("error in (no error)"=w291, "specific error code to clear (0: all)"=w290) -> ("error out"=w298:errorcluster)  [unwired: 4 in, 1 out]
            n148 = control-ref of="This VI"() -> (w287:refnum<vi>)
            n149 = call-dynamic "Delacor_lib_QMH_Release Message Queue.vi"("error in (no error)"=w298, "Message Queue"=w297) -> ("error out"=w294:errorcluster)  [unwired: 9 in]
            n150 = call "Handle Exit.vi"("Stop Argument"=w288, "Admin in"=w286, "VI reference"=w287) -> ("error out"=w285:errorcluster)  [unwired: 7 in, 1 out]
            n151 = call "Application Exit.vi"() -> ("error out"=w284:errorcluster)  [unwired: 11 in]
            n152 = Merge Errors(w285, w284, w294) -> (w293:errorcluster)
          }
          frame Default {
            # "#DQMH_HowTo When the developer created this DQMH Module this case was already part of the module"
            # "'Default' case only runs if there is a message that isn't defined in any of the other cases.  Output a programming error."
            n153 = call "Module Name--constant.vi"() -> ("Module Name"=w300:string)  [unwired: 11 in]
            n154 = xnode ("Error Ring")("parameter 0"=w301, "parameter 1"=w300) -> ("error out"=w302:errorcluster)
          }
        }
        n155 = call-dynamic "Delacor_lib_QMH_Error Handler - Message Handling Loop.vi"("error in (no error)"=w153, "Message Queue in"=w144) -> ("dup error in"=w143:errorcluster)  [unwired: 8 in, 1 out]
      }
    }
    frame Error {
      # "Synchronize Caller Events.vi will inform Start Module.vi that the module has launched and will let the code calling Start Module.vi register for broadcasts and would permit the caller receive the broadcast that an error occurred at launch time."
      n156 = call "Synchronize Caller Events.vi"("Singleton Module Admin in"=w315) -> ("error out"=w312:errorcluster)  [unwired: 9 in, 1 out]
      n157 = call "Module Name--constant.vi"() -> ("Module Name"=w318:string)  [unwired: 11 in]
      n158 = Format Into String(format string="An error occurred during initialization. %s is no longer running.", w318) -> (resulting string=w316:string)  [unwired: 2 in, 1 out]
      n159 = Merge Errors(w314, w312) -> (w313:errorcluster)
      n160 = call "Error Reported.vi"("Additional Information"=w316, "Error"=w313) -> ()  [unwired: 9 in, 1 out]
    }
  }
  n161 = Merge Errors(w7, w16) -> (w6:errorcluster)
  n162 = call "Close Module.vi"("error in (no error)"=w6, "Module Admin in"=w17) -> ("error out"=w9:errorcluster, "External Launch"=w4:bool, "Module Admin out"=w8:refnum<class "Delacor_lib_QMH_Module Admin.lvclass">)  [unwired: 7 in]
  n163 = Unregister For Events(event registration refnum=w14, error in=w9) -> (error out=w5:errorcluster)
  "error out" <- w5
  n164 = case "External Launch?" shown="True" w4 {
    tunnel: w5 -> [_ w320]
    frame False {
    }
    frame True {
      n165 = case shown="No Error" w320 {
        frame No Error {
          n166 = invoke on="Invoke Node" class="VI" method="FP.Close"() -> ()  [unwired: 3 in, 3 out]
        }
        frame Error {
          n167 = invoke on="Invoke Node" class="VI" method="FP.Open"("Activate"=TRUE ("Activate?")) -> ()  [unwired: 4 in, 5 out]
        }
      }
    }
  }
  n168 = local write "Module Admin"(w8) -> ()
